vi "FRCts20_Backend_Comment_PD_reform.vi"(7 "Notes":T1, 8 "error in (no error)":errorcluster, 10 "rows affected 2":i32, 11 "rows affected":i32) -> (0 "error out":errorcluster, 3 "data string":string)   [LabVIEW 2014, in "FRCts20_Backend_Engine.lvlib"]
doc: "Returns whether a comment was successfully updated or deleted"
uses:
  FRCts20_Backend_Engine.lvlib
  FRCts20_Backend_API/Notes.ctl
  FRCts20_Backend_API/ApiReturn.ctl
  FRCts20_Backend_API/NotesRoot.ctl
  FRCts20_Backend_API/FRCts20_Backend_API.lvlib
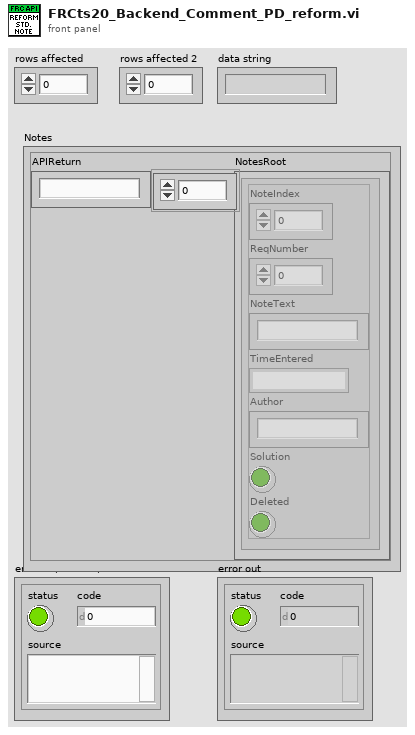
[diagram p1: front panel]
types:
  T1 = typedef "FRCts20_Backend_Engine.lvlib/FRCts20_Backend_API.lvlib/Notes.ctl" = cluster{"APIReturn":T2, "NotesRoot":T3}
  T2 = typedef "FRCts20_Backend_Engine.lvlib/FRCts20_Backend_API.lvlib/ApiReturn.ctl" = string
  T3 = typedef "FRCts20_Backend_Engine.lvlib/FRCts20_Backend_API.lvlib/NotesRoot.ctl" = cluster{"NoteIndex":u32, "ReqNumber":i32, "NoteText":string, "TimeEntered":string, "Author":string, "Solution":bool, "Deleted":bool}[]
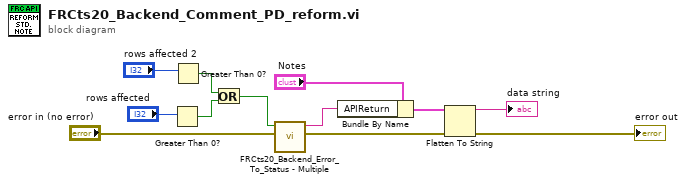
[diagram p0: block diagram]
diagram:
  n1 = Greater Than 0?(x="rows affected") -> (x > 0?=w2:bool)
  n2 = Greater Than 0?(x="rows affected 2") -> (x > 0?=w3:bool)
  n3 = Or(x=w3, y=w2) -> (x .or. y?=w1:bool)
  n4 = call "FRCts20_Backend_Error_To_Status - Multiple.vi"("error in (no error)"="error in (no error)", "rows affected?"=w1) -> ("error out"=w9:errorcluster, "String"=w10:string)  [unwired: 8 in]
  n5 = Bundle By Name(cluster="Notes", "APIReturn"=w10) -> (w7:T1)
  n6 = Flatten To String(anything=w7, error in (no error)=w9) -> (data string=→"data string":string, error out=→"error out":errorcluster)  [unwired: 2 in, 1 out]
